vi "Configure IF Bandwith.vi"(8 "error in (no error)":errorcluster, 10 "IF BW [Hz]":dbl, 11 "VNA-PNA in":refnum<class "VNA-PNA.lvclass">) -> (0 "error out":errorcluster, 2 "IF BW used [Hz]":dbl, 3 "VNA-PNA out":refnum<class "VNA-PNA.lvclass">)   [LabVIEW 2020, in "VNA-PNA.lvclass"]
doc: "Configures the Intermidiate Frequency Bandwidth. \nIt chooses the closest supported bandwidth.\nIt returns the used IF BW."
uses:
  VNA-PNA.lvclass
  C:/Sandbox/Git_Sandbox/WiSpry Test Framework source code (LV20)/WiSpry Test Framework/Instruments/Instrument.lvclass
  C:/Sandbox/Git_Sandbox/WiSpry Test Framework source code (LV20)/WiSpry Test Framework/Instruments/Vector Network Analyzer/Vector Network Analyzer.lvclass
  Instrument.lvclass/Instrument.ctl
  Vector Network Analyzer.lvclass/Vector Network Analyzer.ctl
  Instrument.lvclass
  Vector Network Analyzer.lvclass
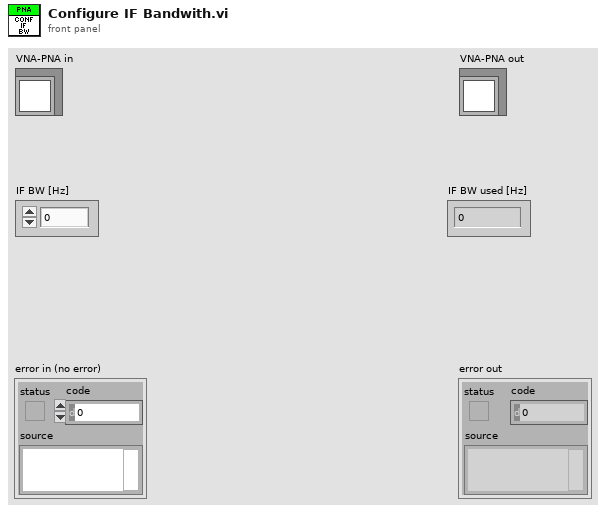
[diagram p1: front panel]
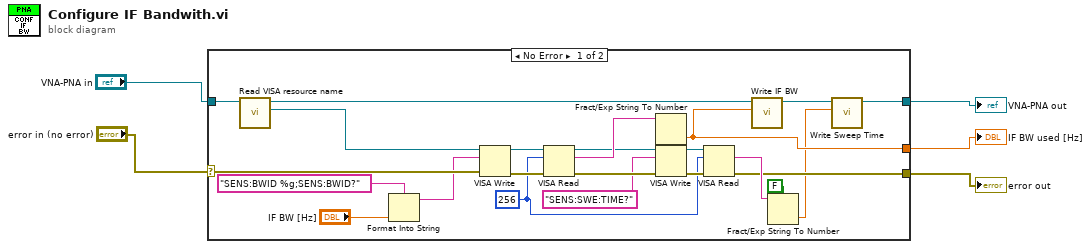
[diagram p0: block diagram]
diagram:
  n1 = case shown="No Error" "error in (no error)" {
    selector: "error in (no error)" -> [w26 w30]
    tunnel: "VNA-PNA in" -> [w28 w29]
    tunnel: [w11 w29] -> w3
    tunnel: [w19 _] -> w2
    tunnel: [w9 w30] -> w1
    frame No Error {
      w13 = u32 256 ("byte count")
      n2 = call "Read VISA resource name.vi"("Instrument in"=w28) -> ("VISA resource name"=w25:refnum<visa-resource-name>, "Instrument out"=w20:refnum<class "VNA-PNA.lvclass">)  [unwired: 9 in]
      n3 = Format Into String(format string="SENS:BWID %g;SENS:BWID?", "IF BW [Hz]") -> (resulting string=w24:string)  [unwired: 2 in, 1 out]
      n4 = VISA Write(VISA resource name=w25, write buffer=w24, error in (no error)=w26) -> (VISA resource name out=w22:refnum<visa-resource-name>, error out=w23:errorcluster)  [unwired: 1 out]
      n5 = VISA Read(VISA resource name=w22, byte count=w13, error in (no error)=w23) -> (VISA resource name out=w17:refnum<visa-resource-name>, read buffer=w21:string, error out=w18:errorcluster)  [unwired: 1 out]
      n6 = Fract/Exp String To Number(string=w21) -> (number=w19:dbl)  [unwired: 3 in, 1 out]
      n7 = VISA Write(VISA resource name=w17, write buffer="SENS:SWE:TIME?", error in (no error)=w18) -> (VISA resource name out=w14:refnum<visa-resource-name>, error out=w15:errorcluster)  [unwired: 1 out]
      n8 = VISA Read(VISA resource name=w14, byte count=w13, error in (no error)=w15) -> (read buffer=w10:string, error out=w9:errorcluster)  [unwired: 2 out]
      n9 = call "Write IF BW.vi"("IF BW"=w19, "Vector Network Analyzer in"=w20) -> ("Vector Network Analyzer out"=w12:refnum<class "VNA-PNA.lvclass">)  [unwired: 9 in]
      n10 = Fract/Exp String To Number(use system decimal point (T)=FALSE, string=w10) -> (number=w8:dbl)  [unwired: 2 in, 1 out]
      n11 = call "Write Sweep Time.vi"("Sweep Time"=w8, "Vector Network Analyzer in"=w12) -> ("Vector Network Analyzer out"=w11:refnum<class "VNA-PNA.lvclass">)  [unwired: 9 in]
    }
    frame Error {
    }
  }
  "error out" <- w1
  "VNA-PNA out" <- w3
  "IF BW used [Hz]" <- w2
